vi "HFRR ADV v036 new software.vi"() -> ()   [LabVIEW 2025] (continued)
          tunnel: [T19."Disabled" ("Disabled") T19."Enabled" ("Disabled")] -> w1363
          frame False {
          }
          frame True {
          }
        }
        n1483 = property on="About" class="Bool (strict)"("DisabledEnum"=w1363) -> ()  [unwired: 2 in, 2 out]
      }
      frame "Test Setup" {
        w1369 = T19."Enabled" ("Disabled")
        n1484 = local read "Service Password enable"() -> (w1368:bool)
        n1485 = property on="Dashboard" class="Bool (strict)"("DisabledEnum"=T19."Disabled" ("Disabled")) -> ()  [unwired: 2 in, 2 out]
        n1486 = property on="Imaging" class="Bool (strict)"("DisabledEnum"=w1369) -> ()  [unwired: 2 in, 2 out]
        n1487 = property on="Analysis" class="Bool (strict)"("DisabledEnum"=w1369) -> ()  [unwired: 2 in, 2 out]
        n1488 = property on="Home" class="Bool (strict)"("DisabledEnum"=w1369) -> ()  [unwired: 2 in, 2 out]
        n1489 = property on="Report" class="Bool (strict)"("DisabledEnum"=w1369) -> ()  [unwired: 2 in, 2 out]
        n1490 = property on="Test Setup" class="Bool (strict)"("DisabledEnum"=w1369) -> ()  [unwired: 2 in, 2 out]
        n1491 = case shown="True" w1368 {
          tunnel: [T19."Disabled" ("Disabled") T19."Enabled" ("Disabled")] -> w1367
          frame False {
          }
          frame True {
          }
        }
        n1492 = property on="About" class="Bool (strict)"("DisabledEnum"=w1367) -> ()  [unwired: 2 in, 2 out]
      }
      frame "Adv Scar" {
        w1376 = T19."Enabled" ("Disabled")
        n1493 = property on="Dashboard" class="Bool (strict)"("DisabledEnum"=T19."Disabled" ("Disabled")) -> ()  [unwired: 2 in, 2 out]
        n1494 = property on="Imaging" class="Bool (strict)"("DisabledEnum"=w1376) -> ()  [unwired: 2 in, 2 out]
        n1495 = property on="Analysis" class="Bool (strict)"("DisabledEnum"=w1376) -> ()  [unwired: 2 in, 2 out]
        n1496 = property on="Home" class="Bool (strict)"("DisabledEnum"=w1376) -> ()  [unwired: 2 in, 2 out]
        n1497 = property on="Report" class="Bool (strict)"("DisabledEnum"=w1376) -> ()  [unwired: 2 in, 2 out]
        n1498 = property on="Test Setup" class="Bool (strict)"("DisabledEnum"=w1376) -> ()  [unwired: 2 in, 2 out]
        n1499 = local read "Service Password enable"() -> (w1374:bool)
        n1500 = case shown="True" w1374 {
          tunnel: [T19."Disabled" ("Disabled") T19."Enabled" ("Disabled")] -> w1373
          frame False {
          }
          frame True {
          }
        }
        n1501 = property on="About" class="Bool (strict)"("DisabledEnum"=w1373) -> ()  [unwired: 2 in, 2 out]
      }
      frame "Calibration" {
        w1379 = T19."Enabled" ("Disabled")
        n1502 = property on="Dashboard" class="Bool (strict)"("DisabledEnum"=T19."Disabled" ("Disabled")) -> ()  [unwired: 2 in, 2 out]
        n1503 = property on="Imaging" class="Bool (strict)"("DisabledEnum"=w1379) -> ()  [unwired: 2 in, 2 out]
        n1504 = property on="Analysis" class="Bool (strict)"("DisabledEnum"=w1379) -> ()  [unwired: 2 in, 2 out]
        n1505 = property on="Home" class="Bool (strict)"("DisabledEnum"=w1379) -> ()  [unwired: 2 in, 2 out]
        n1506 = property on="Report" class="Bool (strict)"("DisabledEnum"=w1379) -> ()  [unwired: 2 in, 2 out]
        n1507 = property on="Test Setup" class="Bool (strict)"("DisabledEnum"=w1379) -> ()  [unwired: 2 in, 2 out]
        n1508 = local read "Service Password enable"() -> (w1381:bool)
        n1509 = property on="Calibration" class="Bool (strict)"("DisabledEnum"=w1379) -> ()  [unwired: 2 in, 2 out]
        n1510 = case shown="True" w1381 {
          tunnel: [T19."Disabled" ("Disabled") T19."Enabled" ("Disabled")] -> w1380
          frame False {
          }
          frame True {
          }
        }
        n1511 = property on="About" class="Bool (strict)"("DisabledEnum"=w1380) -> ()  [unwired: 2 in, 2 out]
      }
      frame "Adv Scar Report" {
        w1387 = T19."Enabled" ("Disabled")
        n1512 = property on="Dashboard" class="Bool (strict)"("DisabledEnum"=T19."Disabled" ("Disabled")) -> ()  [unwired: 2 in, 2 out]
        n1513 = property on="Imaging" class="Bool (strict)"("DisabledEnum"=w1387) -> ()  [unwired: 2 in, 2 out]
        n1514 = property on="Analysis" class="Bool (strict)"("DisabledEnum"=w1387) -> ()  [unwired: 2 in, 2 out]
        n1515 = property on="Home" class="Bool (strict)"("DisabledEnum"=w1387) -> ()  [unwired: 2 in, 2 out]
        n1516 = property on="Report" class="Bool (strict)"("DisabledEnum"=w1387) -> ()  [unwired: 2 in, 2 out]
        n1517 = property on="Test Setup" class="Bool (strict)"("DisabledEnum"=w1387) -> ()  [unwired: 2 in, 2 out]
        n1518 = local read "Service Password enable"() -> (w1386:bool)
        n1519 = case shown="True" w1386 {
          tunnel: [T19."Disabled" ("Disabled") T19."Enabled" ("Disabled")] -> w1385
          frame False {
          }
          frame True {
          }
        }
        n1520 = property on="About" class="Bool (strict)"("DisabledEnum"=w1385) -> ()  [unwired: 2 in, 2 out]
      }
      frame "Compare Files" {
        w1393 = T19."Enabled" ("Disabled")
        n1521 = local read "Service Password enable"() -> (w1392:bool)
        n1522 = property on="Dashboard" class="Bool (strict)"("DisabledEnum"=T19."Disabled" ("Disabled")) -> ()  [unwired: 2 in, 2 out]
        n1523 = property on="Imaging" class="Bool (strict)"("DisabledEnum"=w1393) -> ()  [unwired: 2 in, 2 out]
        n1524 = property on="Analysis" class="Bool (strict)"("DisabledEnum"=w1393) -> ()  [unwired: 2 in, 2 out]
        n1525 = property on="Home" class="Bool (strict)"("DisabledEnum"=w1393) -> ()  [unwired: 2 in, 2 out]
        n1526 = property on="Report" class="Bool (strict)"("DisabledEnum"=w1393) -> ()  [unwired: 2 in, 2 out]
        n1527 = property on="Test Setup" class="Bool (strict)"("DisabledEnum"=w1393) -> ()  [unwired: 2 in, 2 out]
        n1528 = case shown="True" w1392 {
          tunnel: [T19."Disabled" ("Disabled") T19."Enabled" ("Disabled")] -> w1391
          frame False {
          }
          frame True {
          }
        }
        n1529 = property on="About" class="Bool (strict)"("DisabledEnum"=w1391) -> ()  [unwired: 2 in, 2 out]
      }
      frame "Acquire" {
        n1530 = local read "Service Password enable"() -> (w1398:bool)
        n1531 = property on="Test Setup" class="Bool (strict)"("DisabledEnum"=T19."Disabled" ("Disabled")) -> ()  [unwired: 2 in, 2 out]
        n1532 = local read "Auto Start Test"() -> (w1400:bool)
        n1533 = local read "RUN"() -> (w1402:bool)
        n1534 = case shown="True" w1398 {
          tunnel: [T19."Disabled" ("Disabled") T19."Enabled" ("Disabled")] -> w1399
          frame False {
          }
          frame True {
          }
        }
        n1535 = Or(x=w1402, y=w1400) -> (x .or. y?=w1401:bool)
        n1536 = case shown="True" w1401 {
          tunnel: [T19."Enabled" ("Disabled") T19."Disabled" ("Disabled")] -> w1397
          frame False {
          }
          frame True {
          }
        }
        n1537 = property on="About" class="Bool (strict)"("DisabledEnum"=w1399) -> ()  [unwired: 2 in, 2 out]
        n1538 = property on="Imaging" class="Bool (strict)"("DisabledEnum"=w1397) -> ()  [unwired: 2 in, 2 out]
        n1539 = property on="Dashboard" class="Bool (strict)"("DisabledEnum"=w1397) -> ()  [unwired: 2 in, 2 out]
        n1540 = property on="Analysis" class="Bool (strict)"("DisabledEnum"=w1397) -> ()  [unwired: 2 in, 2 out]
        n1541 = property on="Home" class="Bool (strict)"("DisabledEnum"=w1397) -> ()  [unwired: 2 in, 2 out]
        n1542 = property on="Report" class="Bool (strict)"("DisabledEnum"=w1397) -> ()  [unwired: 2 in, 2 out]
        n1543 = property on="Calibration" class="Bool (strict)"("DisabledEnum"=w1397) -> ()  [unwired: 2 in, 2 out]
      }
      frame "About" {
        n1544 = local read "FILE"() -> (w1416:string)
        n1545 = local read "TEST FILE NAM,E SAVED"() -> (w1409:bool)
        n1546 = call <vilib>:"Trim Whitespace.vi"("string"=w1416) -> ("trimmed string"=w1415:string)  [unwired: 1 in]
        n1547 = local read "Auto Start Test"() -> (w1419:bool)
        n1548 = String Length(string=w1415) -> (length=w1414:i32)
        n1549 = Greater?(x=w1414, y=1) -> (0:w1411:bool)
        n1550 = And(x=w1411, y=w1409) -> (x .and. y?=w1410:bool)
        n1551 = local read "RUN"() -> (w1421:bool)
        n1552 = case shown="True" w1410 {
          tunnel: [T19."Disabled" ("Disabled") T19."Enabled" ("Disabled")] -> w1412
          frame False {
          }
          frame True {
          }
        }
        n1553 = Or(x=w1421, y=w1419) -> (x .or. y?=w1420:bool)
        n1554 = property on="About" class="Bool (strict)"("DisabledEnum"=T19."Enabled" ("Disabled")) -> ()  [unwired: 2 in, 2 out]
        n1555 = case shown="False" w1420 {
          tunnel: [T19."Enabled" ("Disabled") T19."Disabled" ("Disabled")] -> w1418
          frame False {
          }
          frame True {
          }
        }
        n1556 = property on="Dashboard" class="Bool (strict)"("DisabledEnum"=w1412) -> ()  [unwired: 2 in, 2 out]
        n1557 = property on="Test Setup" class="Bool (strict)"("DisabledEnum"=T19."Disabled" ("Disabled")) -> ()  [unwired: 2 in, 2 out]
        n1558 = property on="Imaging" class="Bool (strict)"("DisabledEnum"=w1418) -> ()  [unwired: 2 in, 2 out]
        n1559 = property on="Analysis" class="Bool (strict)"("DisabledEnum"=w1418) -> ()  [unwired: 2 in, 2 out]
        n1560 = property on="Home" class="Bool (strict)"("DisabledEnum"=w1418) -> ()  [unwired: 2 in, 2 out]
        n1561 = property on="Report" class="Bool (strict)"("DisabledEnum"=w1418) -> ()  [unwired: 2 in, 2 out]
      }
    }
    n1562 = local read "Quit"() -> (w1346:bool)
    "Single" <- "Single - Graph"
  }
  n1563 = disable-structure shown="Disabled" {
    disable-tunnel: [w1699 _] -> w42
    disable-tunnel: _ -> [w1698 _]
    frame Disabled {
      n1564 = while {
        tunnel: w1698 -> [_]
        tunnel: [w1700] -> w1699
        tunnel: [w1701] -> _
        i -> [w1701]
        stop <- w1700 stop-if-true
        w1717 = u16 10 items=["1.0"=10, "1.5"=15, "2.0"=20] ("stop bits (10: 1 bit)")
        n1565 = Wait (ms)(milliseconds to wait=u32 10) -> ()  [unwired: 1 out]
        n1566 = call-poly "VISA Configure Serial Port"("VISA resource name"=refnum<visa-resource-name> "ASRL1::INSTR" ("COM PORT"), "timeout (10sec)"=u32 10, "baud rate (9600)"=u32 57600, "data bits (8)"=u16 8, "stop bits (10: 1 bit)"=w1717) -> ("VISA resource name out"=w1703:refnum<visa-resource-name>, "error out"=w1712:errorcluster)  [unwired: 9 in]
        n1567 = VISA Read(VISA resource name=w1703, byte count=u32 2 ("byte count (0)")) -> (read buffer=w1711:string)  [unwired: 1 in, 3 out]
        n1568 = String Subset(string=w1711, offset (0)=0, length (rest)=2 ("length (rest)")) -> (substring=w1710:string)
        n1569 = Match Pattern(string=w1710, regular expression="<>") -> (offset past match=w1707:i32)  [unwired: 1 in, 3 out]
        n1570 = Greater Or Equal?(x=w1707, y=0) -> (x >= y?=w1702:bool)
        n1571 = case shown="True" w1702 {
          tunnel: w1703 -> [_ w1721]
          tunnel: w1712 -> [_ w1720]
          frame False {
          }
          frame True {
            n1572 = VISA Read(VISA resource name=w1721, byte count=u32 32 ("byte count (0)"), error in (no error)=w1720) -> (read buffer=w1719:string)  [unwired: 3 out]
            n1573 = String Subset(string=w1719, offset (0)=0, length (rest)=8 ("length (rest)")) -> (substring=w1723:string)
            n1574 = String Subset(string=w1719, offset (0)=8, length (rest)=8 ("length (rest)")) -> (substring=w1724:string)
            n1575 = Decimal String To Number(string=w1724) -> (number=w1731:i32)  [unwired: 2 in, 1 out]
            n1576 = Decimal String To Number(string=w1723) -> (number=w1727:i32)  [unwired: 2 in, 1 out]
            n1577 = Divide(x=w1731, y=10000) -> ()  [unwired: 1 out]
            n1578 = Divide(x=w1727, y=1000000) -> ()  [unwired: 1 out]
          }
        }
        n1579 = local read "Quit"() -> (w1700:bool)
      }
    }
    frame Enabled {
    }
  }
  n1580 = Tick Count (ms)() -> (millisecond timer value=w4:u32)
  n1581 = while {
    shift-right: [w1777] -> _
    shift-left: w6 -> [w1781]
    shift-right: [w1776] -> _
    shift-left: w5 -> [w1780]
    shift-right: [w1775] -> _
    shift-left: w6 -> [w1779]
    shift-right: [w1774] -> _
    shift-left: w5 -> [w1778]
    shift-right: [w1772] -> _
    shift-left: w4 -> [w1773]
    shift-right: [w1769] -> _
    shift-left: w3 -> [w1770]
    shift-right: [w1768] -> _
    shift-left: w3 -> [w1771]
    shift-right: [w1761] -> _
    shift-left: w3 -> [w1767]
    shift-right: [w1760] -> _
    shift-left: w3 -> [w1766]
    shift-right: [w1759] -> _
    shift-left: w3 -> [w1765]
    shift-right: [w1758] -> _
    shift-left: w3 -> [w1764]
    shift-right: [w1757] -> _
    shift-left: w3 -> [w1763]
    shift-right: [w1756] -> _
    shift-left: w3 -> [w1762]
    shift-right: [w1755] -> _
    shift-left: w3 -> [w1749]
    shift-right: [w1754] -> _
    shift-left: w3 -> [w1748]
    shift-right: [w1753] -> _
    shift-left: w3 -> [w1747]
    shift-right: [w1752] -> _
    shift-left: w3 -> [w1746]
    shift-right: [w1751] -> _
    shift-left: w3 -> [w1745]
    shift-right: [w1750] -> _
    shift-left: w3 -> [w1744]
    shift-right: [w1735] -> _
    shift-left: w3 -> [w1738]
    shift-right: [w1734] -> _
    shift-left: w3 -> [w1737]
    shift-right: [w1733] -> _
    shift-left: w3 -> [w1736]
    stop <- w1783 stop-if-true
    n1582 = local read "Read UNO"() -> (w1742:string)
    n1583 = local read "Error  2"() -> (w1782:errorcluster)
    n1584 = String Length(string=w1742) -> (length=w1741:i32)
    n1585 = call <vilib>:"Trim Whitespace.vi"("string"=w1742) -> ("trimmed string"=w1743:string)  [unwired: 1 in]
    n1586 = Greater Or Equal?(x=w1741, y=23) -> (x >= y?=w1739:bool)
    n1587 = case shown="No Error" w1782 {
      tunnel: w1781 -> [w1829 w1925]
      tunnel: w1780 -> [w1828 w1924]
      tunnel: w1779 -> [w1827 w1923]
      tunnel: w1778 -> [w1826 w1922]
      tunnel: [w1825 w1925] -> w1777
      tunnel: [w1824 w1924] -> w1776
      tunnel: [w1823 w1923] -> w1775
      tunnel: [w1822 w1922] -> w1774
      tunnel: w1773 -> [w1821 w1921]
      tunnel: [w1820 w1921] -> w1772
      tunnel: w1770 -> [w1819 w1920]
      tunnel: w1771 -> [w1818 w1919]
      tunnel: [w1817 w1920] -> w1769
      tunnel: [w1816 w1919] -> w1768
      tunnel: w1767 -> [w1815 w1918]
      tunnel: w1766 -> [w1814 w1917]
      tunnel: w1765 -> [w1813 w1916]
      tunnel: w1764 -> [w1812 w1915]
      tunnel: w1763 -> [w1811 w1914]
      tunnel: w1762 -> [w1810 w1913]
      tunnel: [w1809 w1918] -> w1761
      tunnel: [w1808 w1917] -> w1760
      tunnel: [w1807 w1916] -> w1759
      tunnel: [w1806 w1915] -> w1758
      tunnel: [w1805 w1914] -> w1757
      tunnel: [w1804 w1913] -> w1756
      tunnel: w1749 -> [w1803 w1912]
      tunnel: [w1802 w1912] -> w1755
      tunnel: [w1801 w1908] -> w1754
      tunnel: [w1800 w1907] -> w1753
      tunnel: [w1799 w1911] -> w1752
      tunnel: [w1798 w1910] -> w1751
      tunnel: [w1797 w1909] -> w1750
      tunnel: w1748 -> [w1796 w1911]
      tunnel: w1747 -> [w1795 w1910]
      tunnel: w1746 -> [w1794 w1909]
      tunnel: w1745 -> [w1793 w1908]
      tunnel: w1744 -> [w1792 w1907]
      tunnel: w1743 -> [w1791 _]
      tunnel: w1739 -> [w1790 _]
      tunnel: w1738 -> [w1789 w1906]
      tunnel: w1737 -> [w1788 w1905]
      tunnel: w1736 -> [w1787 w1904]
      tunnel: [w1786 w1906] -> w1735
      tunnel: [w1785 w1905] -> w1734
      tunnel: [w1784 w1904] -> w1733
      frame No Error {
        n1588 = case shown="True" w1790 {
          tunnel: w1829 -> [w1845 w1897]
          tunnel: w1828 -> [w1844 w1896]
          tunnel: w1827 -> [w1843 w1895]
          tunnel: w1826 -> [w1842 w1894]
          tunnel: [w1845 w1893] -> w1825
          tunnel: [w1844 w1892] -> w1824
          tunnel: [w1843 w1891] -> w1823
          tunnel: [w1842 w1890] -> w1822
          tunnel: w1821 -> [w1841 w1888]
          tunnel: [w1841 w1887] -> w1820
          tunnel: w1819 -> [w1840 w1886]
          tunnel: w1818 -> [w1839 w1885]
          tunnel: [w1840 w1884] -> w1817
          tunnel: [w1839 w1883] -> w1816
          tunnel: w1815 -> [w1838 w1882]
          tunnel: w1814 -> [w1837 w1881]
          tunnel: w1813 -> [w1836 w1880]
          tunnel: w1812 -> [w1835 w1879]
          tunnel: w1811 -> [w1834 w1878]
          tunnel: w1810 -> [w1833 w1877]
          tunnel: [w1838 w1876] -> w1809
          tunnel: [w1837 w1875] -> w1808
          tunnel: [w1836 w1874] -> w1807
          tunnel: [w1835 w1873] -> w1806
          tunnel: [w1834 w1872] -> w1805
          tunnel: [w1833 w1871] -> w1804
          tunnel: w1803 -> [w1851 w1870]
          tunnel: [w1851 w1869] -> w1802
          tunnel: [w1848 w1868] -> w1801
          tunnel: [w1847 w1867] -> w1800
          tunnel: [w1850 w1866] -> w1799
          tunnel: [w1846 w1865] -> w1798
          tunnel: [w1849 w1864] -> w1797
          tunnel: w1796 -> [w1850 w1863]
          tunnel: w1795 -> [w1849 w1862]
          tunnel: w1794 -> [w1848 w1861]
          tunnel: w1793 -> [w1847 w1860]
          tunnel: w1792 -> [w1846 w1859]
          tunnel: w1791 -> [_ w1858]
          tunnel: w1789 -> [w1832 w1857]
          tunnel: w1788 -> [w1831 w1856]
          tunnel: w1787 -> [w1830 w1855]
          tunnel: [w1832 w1854] -> w1786
          tunnel: [w1831 w1853] -> w1785
          tunnel: [w1830 w1852] -> w1784
          frame False {
          }
          frame True {
            n1589 = Tick Count (ms)() -> (millisecond timer value=w1889:u32)
            n1590 = String To Byte Array(string=w1858) -> (unsigned byte array=w1902:u8[])
            n1591 = Array Size(array=w1902) -> (size(s)=w1901:i32)
            n1592 = formula code="// --- INTERNAL VARIABLE DECLARATIONS ---\nint i = 0;\nint k = 0;\nint start_idx = -1;\nint end_idx = -1;\nint phase = 0;\nint sign0 = 1;\nint sign1 = 1;\nint ch0_val = 0;   \nint ch1_val = 0;   \nfloat ch0_raw = 0.0;\nfloat ch1_raw = 0.0;\nfloat temp0 = 0.0;\nfloat temp1 = 0.0;\nfloat ch0_clean = 0.0;\nfloat ch1_clean = 0.0;\n\nint valid_samples = 0; // FIX: Track if we actually parsed new data this window\nfloat max_allowed_bits = 8388607.0; // FIX: Change this to match your ADC max value\n\n// Temporal intermediate variables for calculation smoothing\nfloat raw_p2p_v = 0.0;\nfloat raw_friction = 0.0;\nfloat raw_cof = 0.0;\n\n// Temporal intermediate variables for Piezo voltage translations\nfloat piezo_min_v = 0.0;\nfloat piezo_max_v = 0.0;\n\n// Initialize output variables to current shift register states right away\nout_LVDT_Min_V = in_LVDT_Min_V;\nout_LVDT_Max_V = in_LVDT_Max_V;\nout_LVDT_P2P_V = in_LVDT_P2P_V;\nout_Piezo_P2P = in_Piezo_P2P;\nout_Friction_N = in_Friction_N;\nout_COF = in_COF;\nwindow_ready = 0;\n\n// --- STEP 1: PARSE EVERY STRING IN THE BYTE ARRAY ---\nif (array_size > 2) {\n    for (i = 0; i < array_size - 1; i++) {\n        if (raw_bytes[i] == 42) { // '*' character detected\n            start_idx = i;\n        }\n        \n        // Match standard delimiter sequence \";&\" or end window character\n        if (raw_bytes[i] == 59 && raw_bytes[i+1] == 38 && start_idx != -1) { \n            end_idx = i;\n            ch0_val = 0;\n            ch1_val = 0;\n            sign0 = 1;\n            sign1 = 1;\n            phase = 0; \n\n            for (k = start_idx + 1; k < end_idx; k++) {\n                if (raw_bytes[k] == 45) { // '-' sign\n                    if (phase == 0) sign0 = -1;\n                    else sign1 = -1;\n                }\n                else if (raw_bytes[k] == 43) { // '+' sign\n                    if (phase == 0) sign0 = 1;\n                    else sign1 = 1;\n                }\n                else if (raw_bytes[k] == 59) { // ';' delimiter\n                    phase = 1; \n                }\n                else if (raw_bytes[k] >= 48 && raw_bytes[k] <= 57) { // Numeric ASCII digits\n                    if (phase == 0) {\n                        ch0_val = (ch0_val * 10) + (raw_bytes[k] - 48);\n                    } else {\n                        ch1_val = (ch1_val * 10) + (raw_bytes[k] - 48);\n                    }\n                }\n            }\n\n            // Implicit type conversion\n            ch0_raw = ch0_val * sign0 * 1.0;\n            ch1_raw = ch1_val * sign1 * 1.0;\n\n            // FIX: Sanity check / Hard-clamping to catch sudden massive ASCII noise spikes\n            if (ch0_raw > max_allowed_bits)  ch0_raw = max_allowed_bits;\n            if (ch0_raw < -max_allowed_bits) ch0_raw = -max_allowed_bits;\n            if (ch1_raw > max_allowed_bits)  ch1_raw = max_allowed_bits;\n            if (ch1_raw < -max_allowed_bits) ch1_raw = -max_allowed_bits;\n\n            // --- STEP 2: 3-SAMPLE MEDIAN FILTER ---\n            m0_2 = m0_1; m0_1 = m0_0; m0_0 = ch0_raw;\n            float s0_0 = m0_0; float s0_1 = m0_1; float s0_2 = m0_2;\n            if (s0_0 > s0_1) { temp0 = s0_0; s0_0 = s0_1; s0_1 = temp0; }\n            if (s0_1 > s0_2) { temp0 = s0_1; s0_1 = s0_2; s0_2 = temp0; }\n            if (s0_0 > s0_1) { temp0 = s0_0; s0_0 = s0_1; s0_1 = temp0; }\n            ch0_clean = s0_1;\n\n            m1_2 = m1_1; m1_1 = m1_0; m1_0 = ch1_raw;\n            float s1_0 = m1_0; float s1_1 = m1_1; float s1_2 = m1_2;\n            if (s1_0 > s1_1) { temp1 = s1_0; s1_0 = s1_1; s1_1 = temp1; }\n            if (s1_1 > s1_2) { temp1 = s1_1; s1_1 = s1_2; s1_2 = temp1; }\n            if (s1_0 > s1_1) { temp1 = s1_0; s1_0 = s1_1; s1_1 = temp1; }\n            ch1_clean = s1_1;\n\n            // --- STEP 3: EXPONENTIAL FILTER (STREAM LEVEL) ---\n            if (ch0_filt == 0.0) ch0_filt = ch0_clean;\n            if (ch1_filt == 0.0) ch1_filt = ch1_clean;\n\n            ch0_filt = ch0_filt + (ch0_clean - ch0_filt) * 0.125;\n            ch1_filt = ch1_filt + (ch1_clean - ch1_filt) * 0.125;\n\n            // --- STEP 4: MIN/MAX WINDOW CONTINUOUS ACCUMULATION ---\n            if (ch0_filt > max_ch0) max_ch0 = ch0_filt;\n            if (ch0_filt < min_ch0) min_ch0 = ch0_filt;\n            if (ch1_filt > max_ch1) max_ch1 = ch1_filt;\n            if (ch1_filt < min_ch1) min_ch1 = ch1_filt;\n\n            valid_samples++; // FIX: Successfully parsed and accumulated a clean point\n            start_idx = -1; \n        }\n    }\n}\n\n// --- STEP 5: WINDOW EVALUATION ENGINE ---\n// FIX: Condition updated to verify that valid samples exist for both channels\nif (((current_time_ms - start_time_ms) >= 50) && (valid_samples > 0) && (min_ch0 < 9000000.0) && (min_ch1 < 9000000.0)) {\n    window_ready = 1;\n\n    // Linear Bit-to-Voltage Transformations (LVDT - Channel 0)\n    out_LVDT_Min_V = (min_ch0 * VREF) / 8388607.0;\n    out_LVDT_Max_V = (max_ch0 * VREF) / 8388607.0;\n    raw_p2p_v = out_LVDT_Max_V - out_LVDT_Min_V;\n\n    // Linear Bit-to-Voltage Transformations (Piezo - Channel 1)\n    piezo_min_v = (min_ch1 * VREF) / 8388607.0;\n    piezo_max_v = (max_ch1 * VREF) / 8388607.0;\n    \n    // Assign Peak-to-Peak Voltage directly to output indicator (Matches Python logic)\n    out_Piezo_P2P = piezo_max_v - piezo_min_v;\n    \n    // Force scaling calculations using Voltage delta * Newtons/Volt Factor\n    raw_friction = out_Piezo_P2P * PIEZO_CAL_FACTOR + 0.44528;\n    raw_cof = raw_friction / NORMAL_FORCE;\n\n    // --- STEP 6: OUTPUT METRIC SMOOTHING (Low-Pass Filter Alpha = 0.05) ---\n    // Seed initial historical metrics if first loop iteration\n    if (hist_LVDT_P2P == 0.0) hist_LVDT_P2P = raw_p2p_v;\n    if (hist_Friction == 0.0) hist_Friction = raw_friction;\n    if (hist_COF == 0.0)      hist_COF = raw_cof;\n\n    // Apply exponential output dampening\n    hist_LVDT_P2P = hist_LVDT_P2P + (raw_p2p_v - hist_LVDT_P2P) * 0.05;\n    hist_Friction = hist_Friction + (raw_friction - hist_Friction) * 0.05; // Note: Can drop to 0.02 for more aggressive damping\n    hist_COF      = hist_COF + (raw_cof - hist_COF) * 0.05;\n\n    // Direct smoothed parameters out to UI Indicators\n    out_LVDT_P2P_V = hist_LVDT_P2P;\n    out_Friction_N = hist_Friction;\n    out_COF        = hist_COF;\n\n    // Reset tracking targets to extreme boundaries safely\n    min_ch0 = 9999999.0;\n    max_ch0 = -9999999.0;\n    min_ch1 = 9999999.0;\n    max_ch1 = -9999999.0;\n\n    valid_samples = 0; // FIX: Reset counter for next time frame\n    start_time_ms = current_time_ms;\n}"("raw_bytes"=w1902, "array_size"=w1901, "VREF"="VREF", "PIEZO_CAL_FACTOR"="PIEZO_CAL_FACTOR", "NORMAL_FORCE"="NORMAL_FORCE", "min_ch0"=w1897, "max_ch0"=w1896, "min_ch1"=w1895, "max_ch1"=w1894, "current_time_ms"=w1889, "start_time_ms"=w1888, "ch0_filt"=w1886, "ch1_filt"=w1885, "m0_0"=w1882, "m0_1"=w1881, "m0_2"=w1880, "m1_0"=w1879, "m1_1"=w1878, "m1_2"=w1877, "in_LVDT_Min_V"=w1870, "in_LVDT_Max_V"=w1863, "in_LVDT_P2P_V"=w1862, "in_Piezo_P2P"=w1861, "in_Friction_N"=w1860, "in_COF"=w1859, "hist_LVDT_P2P"=w1857, "hist_Friction"=w1856, "hist_COF"=w1855) -> ("window_ready"=→"Valid_data":dbl, "out_LVDT_Min_V"=w1869:dbl, "out_LVDT_Max_V"=w1868:dbl, "out_LVDT_P2P_V"=w1867:dbl, "out_Piezo_P2P"=w1866:dbl, "out_Friction_N"=w1865:dbl, "out_COF"=w1864:dbl, "min_ch0"=w1893:dbl, "max_ch0"=w1892:dbl, "min_ch1"=w1891:dbl, "max_ch1"=w1890:dbl, "start_time_ms"=w1887:u32, "ch0_filt"=w1884:dbl, "ch1_filt"=w1883:dbl, "m0_0"=w1876:dbl, "m0_1"=w1875:dbl, "m0_2"=w1874:dbl, "m1_0"=w1873:dbl, "m1_1"=w1872:dbl, "m1_2"=w1871:dbl, "hist_LVDT_P2P"=w1854:dbl, "hist_Friction"=w1853:dbl, "hist_COF"=w1852:dbl)
            "LVDT MIN" <- w1869
            "LVDT MAX" <- w1868
            "LVDT Peak" <- w1867
            "pizo raw" <- w1866
            "cof" <- w1864
            "Frictioin Force Raw" <- w1865
          }
        }
      }
      frame Error {
      }
    }
    n1593 = local read "Quit"() -> (w1783:bool)
  }
  n1594 = disable-structure shown="Disabled" {
    disable-tunnel: errorcluster {"status"=TRUE, "code"=0, "source"="Init"} ("error IO") -> [w1928 _]
    disable-tunnel: [w1926 _] -> w45
    frame Disabled {
      n1595 = while {
        shift-right: [w1944] -> w1930
        shift-left: _ -> [w1935]
        shift-right: [w1943] -> w1929
        shift-left: w1928 -> [w1937]
        tunnel: [w1932] -> w1926
        tunnel: [w1942] -> _
        i -> [w1942]
        stop <- w1932 stop-if-true
        n1596 = local read "Port 1a"() -> (w1938:bool)
        n1597 = local read "Port 3"() -> (w1939:bool)
        n1598 = local read "Com Port 1"() -> (w1936:refnum<visa-resource-name>)
        n1599 = Or(x=w1939, y=w1938) -> (x .or. y?=w1941:bool)
        n1600 = Unbundle(w1937) -> ("status"=→"Port 3":bool)  [unwired: 2 out]
        n1601 = Not Equal?(x=w1936, y=w1935) -> (x != y?=w1933:bool)
        n1602 = case shown="True" w1941 {
          frame False {
            w1947 = TRUE ("Visible")
            n1603 = property on="Port 1a" class="Bool (strict)"("Visible"=w1947) -> ()  [unwired: 2 in, 2 out]
            n1604 = property on="Port 3" class="Bool (strict)"("Visible"=w1947) -> ()  [unwired: 2 in, 2 out]
          }
          frame True {
            w1948 = TRUE ("Visible")
            n1605 = property on="Port 1a" class="Bool (strict)"("Visible"=w1948) -> ()  [unwired: 2 in, 2 out]
            n1606 = property on="Port 3" class="Bool (strict)"("Visible"=w1948) -> ()  [unwired: 2 in, 2 out]
          }
        }
        n1607 = Wait (ms)(milliseconds to wait=u32 40) -> ()  [unwired: 1 out]
        n1608 = case shown="True" w1933 {
          tunnel: [w1945 errorcluster {"status"=TRUE, "code"=0, "source"="Init"} ("error out")] -> w1934
          tunnel: w1937 -> [w1945 _]
          frame False {
          }
          frame True {
          }
        }
        n1609 = case shown="Error" w1934 {
          selector: w1934 -> [w1955 w1973]
          tunnel: [w1958 w1977] -> w1944
          tunnel: [w1957 w1971] -> w1943
          tunnel: w1935 -> [w1956 w1975]
          frame No Error {
            n1610 = property class="Instr"(reference=w1956, error in=w1955) -> (reference out=w1953:refnum<visa-resource-name>, error out=w1954:errorcluster, "Serial Settings:Number of Bytes at Serial Port"=w1950:u32)
            n1611 = Greater?(x=w1950, y=u32 5) -> (0:w1949:bool)
            n1612 = Not(x=w1949) -> (.not. x?=→"Port 1a":bool)
            n1613 = while {
              tunnel: [w1966] -> w1957
              tunnel: [w1965] -> w1958
              tunnel: w1954 -> [w1964]
              tunnel: w1953 -> [w1963]
              stop <- TRUE stop-if-true
              n1614 = property class="Instr" props=["Serial Settings:Number of Bytes at Serial Port"](reference=w1963, error in=w1964) -> (reference out=w1968:refnum<visa-resource-name>, error out=w1967:errorcluster)  [unwired: 1 out]
              n1615 = VISA Read(VISA resource name=w1968, byte count=u32 50, error in (no error)=w1967) -> (VISA resource name out=w1965:refnum<visa-resource-name>, read buffer=w1960:string, error out=w1966:errorcluster)  [unwired: 1 out]
              n1616 = Wait (ms)(milliseconds to wait=u32 5) -> ()  [unwired: 1 out]
            }
          }
          frame Error {
            w1983 = u16 0 items=["None", "XON/XOFF", "RTS/CTS", "XON/XOFF & RTS/CTS", "DTR/DSR", "XON/XOFF & DTR/DSR"] ("flow control (0:none)  2")
            w1981 = u16 10 items=["1.0"=10, "1.5"=15, "2.0"=20] ("stop bits 2")
            w1979 = u16 0 items=["None", "Odd", "Even", "Mark", "Space"] ("parity 2")
            w1980 = u32 10000  # timeout (10sec)
            n1617 = VISA Close(VISA resource name=w1975, error in (no error)=w1973) -> (error out=w1976:errorcluster)
            n1618 = local write "Port 1a"(FALSE ("Port 1a")) -> ()
            n1619 = local read "Com Port 1"() -> (w1970:refnum<visa-resource-name>)
            n1620 = call <vilib>:"Clear Errors.vi"("error in (no error)"=w1976) -> ("error out"=w1974:errorcluster)  [unwired: 5 in, 1 out]
            n1621 = call-poly "VISA Configure Serial Port"("VISA resource name"=w1970, "timeout (10sec)"=w1980, "baud rate (9600)"=u32 250000 ("baud rate  2"), "data bits (8)"=u16 8 ("data bits  2"), "parity (0:none)"=w1979, "error in (no error)"=w1974, "stop bits (10: 1 bit)"=w1981, "flow control (0:none)"=w1983) -> ("VISA resource name out"=w1984:refnum<visa-resource-name>, "error out"=w1985:errorcluster)  [unwired: 6 in]
            n1622 = flat-sequence {
              tunnel: w1984 -> [w1987]
              tunnel: w1985 -> [w1986]
              tunnel: [w1987] -> w1977
              tunnel: [w1986] -> w1971
              frame #0 {
                n1623 = Wait (ms)(milliseconds to wait=u32 50) -> ()  [unwired: 1 out]
              }
            }
            "Residual Uno" <- ""
          }
        }
        n1624 = local read "Quit"() -> (w1932:bool)
        "Error Uno" <- w1937
      }
      n1625 = VISA Close(VISA resource name=w1930, error in (no error)=w1929) -> (error out=w1927:errorcluster)
      n1626 = call <vilib>:"Clear Errors.vi"("error in (no error)"=w1927) -> ()  [unwired: 5 in, 2 out]
    }
    frame Enabled {
    }
  }
  n1627 = while {
    stop <- w1998 stop-if-true
    # "V0OLTAGE TO STROKE (peice vise calibration)"
    n1628 = local read "LVDT MIN"() -> (w1990:dbl)
    n1629 = local read "LVDT Peak"() -> (w1989:dbl)
    n1630 = Wait (ms)(milliseconds to wait=u32 10) -> ()  [unwired: 1 out]
    n1631 = formula code="// Dynamic Parameterized Linear Interpolation Node\n// Inputs: vpp_val, voltages (Array), distances (Array)\n// Outputs: stroke\n\nint i = 0;\nint segments = 11; // 12 points make 11 interpolation segments\n\n// 1. Lower Boundary Clamp\nif (vpp_val <= voltages[0]) {\n    stroke = distances[0];\n}\n// 2. Upper Boundary Clamp\nelse if (vpp_val >= voltages[segments]) {\n    stroke = distances[segments];\n}\n// 3. Dynamic Segment Search Loop\nelse {\n    stroke = distances[0]; // Fallback baseline\n    for (i = 0; i < segments; i++) {\n        if (vpp_val >= voltages[i] && vpp_val <= voltages[i+1]) {\n            // Standard linear interpolation formula using array lookups\n            stroke = distances[i] + (vpp_val - voltages[i]) * (distances[i+1] - distances[i]) / (voltages[i+1] - voltages[i]);\n            break; // Segment found, safely exit the loop\n        }\n    }\n}"("vpp_val"=w1989, "voltages"="calibration values", "distances"="STROKE") -> ("stroke"=→"LVDT STROKE":dbl)
    n1632 = local read "Calibration Tare Value"() -> (w1994:dbl)
    n1633 = local read "Calibration Tare"() -> (w1992:bool)
    n1634 = Subtract(x=w1990, y=w1994) -> (x-y=→"LVDT STROKE  Calibration":dbl)
    n1635 = case shown="True" w1992 {
      selector: w1992 -> [_ w2000]
      tunnel: w1990 -> [_ w2001]
      frame False {
      }
      frame True {
        n1636 = Not(x=w2000) -> (.not. x?=w1999:bool)
        n1637 = local write "Calibration Tare"(w1999) -> ()
        "Calibration Tare Value" <- w2001
      }
    }
    n1638 = local read "Quit"() -> (w1998:bool)
  }
  n1639 = while {
    stop <- w2024 stop-if-true
    n1640 = local read "Due read"() -> (w2022:string)
    n1641 = call <vilib>:"High Resolution Polling Wait.vi"("seconds to wait"=0.02) -> ()  [unwired: 10 in, 1 out]
    n1642 = local read "Frictioin Force Raw"() -> (w2004:dbl)
    n1643 = Spreadsheet String To Array(delimiter (Tab)=";", format string="", spreadsheet string=w2022, array type (2D Dbl)=string[] []) -> (array=w2019:string[])
    n1644 = Fract/Exp String To Number(string=w2019) -> (number=w2018:dbl[])  [unwired: 3 in, 1 out]
    n1645 = call <vilib>:"Median Filter PtByPt.vi"("rank"=2, "x"=w2004) -> ("Filtered x"=→"Friction":dbl)  [unwired: 2 in, 1 out]
    n1646 = Index Array(array=w2018) -> (element #1=→"Sample Temperature":dbl, element #2=→"Target Sample Temperature":dbl, element #3=→"Current Duty Cycle":dbl, element #4=→"Ambient Temperature":dbl, element #5=→"Dac Status":dbl, element #6=→"Vpp":dbl, element #7=→"Active Error Code":dbl, element #8=→"Kp":dbl, element #9=→"Ki":dbl, element #10=→"Kd":dbl, element #11=→"SampleRaw":dbl, element #12=→"AmbRaw":dbl)  [unwired: 12 in]
    n1647 = local read "Quit"() -> (w2024:bool)
  }
  n1648 = while {
    shift-right: [w2038] -> w41
    shift-left: _ -> [w2030]
    shift-right: [w2025] -> w40
    shift-left: errorcluster {"status"=FALSE, "code"=0, "source"="Init"} ("error out") -> [w2032]
    tunnel: [w2027] -> w44
    tunnel: [w2037] -> _
    i -> [w2037]
    stop <- w2027 stop-if-true
    n1649 = local read "Com Port 2"() -> (w2031:refnum<visa-resource-name>)
    n1650 = local read "Port 2a"() -> (w2033:bool)
    n1651 = Unbundle(w2032) -> ("status"=→"Port 4":bool)  [unwired: 2 out]
    n1652 = call <vilib>:"High Resolution Polling Wait.vi"("seconds to wait"=0.02) -> ()  [unwired: 10 in, 1 out]
    n1653 = local read "Port 4"() -> (w2034:bool)
    n1654 = Not Equal?(x=w2031, y=w2030) -> (x != y?=w2029:bool)
    n1655 = Or(x=w2034, y=w2033) -> (x .or. y?=w2036:bool)
    n1656 = case shown="False" w2036 {
      frame False {
        w2041 = TRUE ("Visible")
        n1657 = property on="Port 2a" class="Bool (strict)"("Visible"=w2041) -> ()  [unwired: 2 in, 2 out]
        n1658 = property on="Port 4" class="Bool (strict)"("Visible"=w2041) -> ()  [unwired: 2 in, 2 out]
      }
      frame True {
        w2042 = TRUE ("Visible")
        n1659 = property on="Port 2a" class="Bool (strict)"("Visible"=w2042) -> ()  [unwired: 2 in, 2 out]
        n1660 = property on="Port 4" class="Bool (strict)"("Visible"=w2042) -> ()  [unwired: 2 in, 2 out]
      }
    }
    n1661 = case shown="True" w2029 {
      tunnel: [w2039 errorcluster {"status"=TRUE, "code"=0, "source"="Init"} ("error out")] -> w2028
      tunnel: w2032 -> [w2039 _]
      frame False {
      }
      frame True {
      }
    }
    n1662 = case shown="No Error" w2028 {
      selector: w2028 -> [w2055 w2086]
      tunnel: [w2048 w2091] -> w2038
      tunnel: [w2056 w2084] -> w2025
      tunnel: w2030 -> [w2057 w2089]
      frame No Error {
        n1663 = property class="Instr" props=["Serial Settings:Number of Bytes at Serial Port"](reference=w2057, error in=w2055) -> (reference out=w2049:refnum<visa-resource-name>, error out=w2054:errorcluster)  [unwired: 1 out]
        n1664 = while {
          tunnel: [w2065] -> w2050
          tunnel: [w2064] -> w2051
          tunnel: w2054 -> [w2063]
          tunnel: w2049 -> [w2062]
          tunnel: [w2061] -> _
          i -> [w2061]
          stop <- TRUE stop-if-true
          n1665 = property class="Instr" props=["Serial Settings:Number of Bytes at Serial Port"](reference=w2062, error in=w2063) -> (reference out=w2067:refnum<visa-resource-name>, error out=w2066:errorcluster)  [unwired: 1 out]
          n1666 = VISA Read(VISA resource name=w2067, byte count=u32 1000, error in (no error)=w2066) -> (VISA resource name out=w2064:refnum<visa-resource-name>, read buffer=→"Due read":string, error out=w2065:errorcluster)  [unwired: 1 out]
        }
        n1667 = local read "Due Write"() -> (w2047:string)
        n1668 = call <vilib>:"Trim Whitespace.vi"("string"=w2047) -> ("trimmed string"=w2046:string)  [unwired: 1 in]
        n1669 = Not Equal?(x=w2046, y="") -> (x != y?=w2052:bool)
        n1670 = VISA Flush I/O Buffer(VISA resource name=w2051) -> (VISA resource name out=w2044:refnum<visa-resource-name>, error out=→"error out 10":errorcluster)  [unwired: 2 in]
        n1671 = case shown="True" w2052 {
          tunnel: w2044 -> [w2069 w2074]
          tunnel: [w2069 w2078] -> w2048
          tunnel: w2050 -> [w2068 w2073]
          tunnel: [w2068 w2076] -> w2056
          tunnel: w2046 -> [_ w2072]
          tunnel: [_ w2075] -> _
          frame False {
            # "DATA  WRITE LOOP"
          }
          frame True {
            n1672 = Concatenate Strings(w2072, "\r\n") -> (w2071:string)
            n1673 = VISA Write(VISA resource name=w2074, write buffer=w2071, error in (no error)=w2073) -> (VISA resource name out=w2078:refnum<visa-resource-name>, return count=w2075:u32, error out=w2077:errorcluster)
            n1674 = flat-sequence {
              tunnel: w2077 -> [w2080]
              tunnel: [w2080] -> w2076
              frame #0 {
                n1675 = local write "Due Write"("" ("Command")) -> ()
                n1676 = Wait (ms)(milliseconds to wait=u32 5) -> ()  [unwired: 1 out]
              }
            }
          }
        }
        "Port 2a" <- TRUE ("Port 2a")
      }
      frame Error {
        w2097 = u16 0 items=["None", "XON/XOFF", "RTS/CTS", "XON/XOFF & RTS/CTS", "DTR/DSR", "XON/XOFF & DTR/DSR"] ("flow control (0:none)  2")
        w2095 = u16 10 items=["1.0"=10, "1.5"=15, "2.0"=20] ("stop bits 2")
        w2093 = u16 0 items=["None", "Odd", "Even", "Mark", "Space"] ("parity 2")
        w2094 = u32 10000  # timeout (10sec)
        n1677 = VISA Clear(VISA resource name=w2089, error in (no error)=w2086) -> (VISA resource name out=w2088:refnum<visa-resource-name>, error out=w2087:errorcluster)
        n1678 = VISA Close(VISA resource name=w2088, error in (no error)=w2087) -> (error out=w2090:errorcluster)
        n1679 = call <vilib>:"Clear Errors.vi"("error in (no error)"=w2090) -> ()  [unwired: 5 in, 2 out]
        n1680 = local write "Port 2a"(FALSE ("Port 2a")) -> ()
        n1681 = local read "Com Port 2"() -> (w2083:refnum<visa-resource-name>)
        "visa due" <- w2083
        n1682 = call-poly "VISA Configure Serial Port"("VISA resource name"=w2083, "timeout (10sec)"=w2094, "baud rate (9600)"=u32 250000 ("baud rate  2"), "data bits (8)"=u16 8 ("data bits  2"), "parity (0:none)"=w2093, "stop bits (10: 1 bit)"=w2095, "flow control (0:none)"=w2097) -> ("VISA resource name out"=w2098:refnum<visa-resource-name>, "error out"=w2099:errorcluster)  [unwired: 7 in]
        n1683 = flat-sequence {
          tunnel: w2098 -> [w2101]
          tunnel: w2099 -> [w2100]
          tunnel: [w2101] -> w2091
          tunnel: [w2100] -> w2084
          frame #0 {
            n1684 = Wait (ms)(milliseconds to wait=u32 50) -> ()  [unwired: 1 out]
          }
        }
        "Residual Due" <- ""
      }
    }
    "error out 9" <- w2025
    n1685 = local read "Quit"() -> (w2027:bool)
    "Error Due" <- w2032
  }
  n1686 = local write "FRICVALZ"(0.0 ("FRICVALZ")) -> ()
  n1687 = property on="RUN" class="Bool (strict)"("Visible"=TRUE) -> ()  [unwired: 2 in, 2 out]
  n1688 = while {
    tunnel: [w2116] -> _
    tunnel: [w2103] -> w54
    i -> [w2116]
    stop <- w2103 stop-if-true
    n1689 = local read "conststatus"() -> (w2107:dbl)
    n1690 = local read "Main Tab"() -> (w2105:T2)
    n1691 = local read "EDIT"() -> (w2122:bool)
    n1692 = local read "Rate"() -> (w2121:dbl)
    n1693 = case shown="True" w2122 {
      tunnel: [FALSE TRUE] -> _
      frame False {
      }
      frame True {
      }
    }
    n1694 = Equal?(x=w2105, y=T28."About" ("Main Tab")) -> (x = y?=w2114:bool)
    n1695 = Equal?(x=w2107, y=0.0) -> (x = y?=w2108:bool)
    n1696 = Divide(x=1.0, y=w2121) -> (x/y=w2117:dbl)
    "Time 2" <- w2117
    n1697 = case shown="True" w2108 {
      frame False {
      }
      frame True {
        # "C:\\WinDucom\\calibrate WO 2391.dcf"
        n1698 = local write "Lan flag"(22) -> ()
        n1699 = local write "conststatus"(10.0 ("rpm value : 2")) -> ()
        n1700 = String To Path(string="C:\\LAB-IQ\\calibrate WO 2465.dcf") -> (path=w2128:path)
        n1701 = Open/Create/Replace File "Open File"(file path (use dialog)=w2128) -> (refnum out=w2126:refnum<file>)  [unwired: 5 in, 2 out]
        n1702 = for {
          N: 23 -> [_]
          tunnel: w2126 -> [w2137]
          i -> [w2131]
          (unwired) TRUE ("line mode (F)")
          n1703 = Read from Text File "Read File"(file (use dialog)=w2137) -> (text=w2136:string)  [unwired: 3 in, 3 out]
          n1704 = Match Pattern(string=w2136, regular expression="]") -> (after substring=w2134:string)  [unwired: 1 in, 3 out]
          n1705 = String Subset(string=w2136, offset (0)=5, length (rest)=10 ("length (rest)")) -> (substring=w2129:string)
          n1706 = Fract/Exp String To Number(string=w2129) -> (number=w2130:dbl)  [unwired: 3 in, 1 out]
          n1707 = Match Pattern(string=w2134, regular expression="-") -> (before substring=w2132:string)  [unwired: 1 in, 3 out]
          n1708 = case shown="10" w2131 {
            tunnel: w2130 -> [_ _ _ _ _ _ _ _ _ _ w2144 _ _ _ _ _ _ _ _ _ _ _ _ _]
            tunnel: w2132 -> [_ _ _ _ w2140 w2141 w2142 _ _ _ _ _ _ _ _ _ _ _ _ _ w2145 w2146 w2147 _]
            frame 0 {
            }
            frame 1 {
            }
            frame 2 {
            }
            frame 3 {
            }
            frame 4 {
              n1709 = local write "Com Port 1"(w2140) -> ()
            }
            frame 5 {
              n1710 = local write "Com Port 2"(w2141) -> ()
              n1711 = local write "visa due"(w2141) -> ()
            }
            frame 6 {
              n1712 = String To Path(string=w2142) -> (path=w2143:path)
              n1713 = local write "File Path"(w2143) -> ()
              "String" <- w2142
            }
            frame 7 {
            }
            frame 8 {
            }
            frame 9 {
            }
            frame 10 {
              n1714 = local write "Language Selection"(w2144) -> ()
            }
            frame 11 {
            }
            frame 12 {
            }
            frame 13 {
            }
            frame 14 {
            }
            frame 15 {
            }
            frame 16 {
            }
            frame 17 {
            }
            frame 18 {
            }
            frame 21 {
            }
            frame 22 {
              n1715 = local write "Com Port 3"(w2145) -> ()
            }
            frame 20 {
              n1716 = local write "Camera Port :"(w2146) -> ()
            }
            frame 19 {
              n1717 = local write "C3 :"(w2147) -> ()
            }
            frame 23, Default {
            }
          }
        }
      }
    }
    n1718 = Select(t=u32 2500 ("milliseconds to wait"), s=w2114, f=u32 500 ("milliseconds to wait")) -> (s? t:f=w2112:u32)
    n1719 = Multiply(x=w2117, y=w2112) -> (x*y=w2119:dbl)
    n1720 = call "Elapsed Time2"("Time Target (s)"=w2119, "Auto Reset"=TRUE) -> ("Time has Elapsed"=w2109:bool)  [unwired: 10 in, 7 out]
    n1721 = case shown="True" w2109 {
      frame False {
      }
      frame True {
        n1722 = stacked-sequence {
          frame #0 {
            # "DATA PROCESSING"
            # "115 mV/N"
            n1723 = local read "Sample Temperature"() -> (w2150:dbl)
            n1724 = local read "RH Numeric:"() -> (→"Humidity ( %RH )" →"Hum":dbl)
            n1725 = local read "FRICVALZ"() -> (w2167:dbl)
            n1726 = local read "Friction"() -> (w2153:dbl)
            n1727 = call <vilib>:"Mean PtByPt.vi"("x"=w2150, "sample length"=100) -> ("mean"=w2149:dbl)  [unwired: 2 in, 1 out]
            "TEMP 2" <- w2149
            "TEMP 3" <- w2149
            n1728 = Subtract(x=w2153, y=w2167) -> (x-y=w2162:dbl)
            "FF 2" <- w2162
            "FF 4" <- w2162
            n1729 = local read "Ambient Temperature"() -> (→"AIR TEMP":dbl)
            n1730 = local read "TEMP"() -> (w2166:dbl)
            n1731 = local write "FF 3"(w2162) -> ()
            n1732 = Compound Arithmetic op=OR("FRICVALZ 4", "FRICVALZ 3", "FRICVALZ 2") -> (w2158:bool)
            n1733 = case shown="True" w2158 {
              tunnel: w2153 -> [_ w2173]
              frame False {
              }
              frame True {
                w2172 = FALSE ("FRICVALZ")
                n1734 = local write "FRICVALZ 3"(w2172) -> ()
                n1735 = local write "FRICVALZ 2"(w2172) -> ()
                n1736 = local write "FRICVALZ 4"(w2172) -> ()
                "FRICVALZ" <- w2173
              }
            }
            n1737 = Not A Number/Path/Refnum?(number/path/refnum=w2166) -> (NaN/Path/Refnum?=w2165:bool)
            n1738 = Not A Number/Path/Refnum?(number/path/refnum=w2162) -> (NaN/Path/Refnum?=w2164:bool)
            n1739 = Divide(x=w2162, y=1.96) -> (x/y=w2159:dbl)
            n1740 = Compound Arithmetic op=OR(w2165, w2164) -> (w2163:bool)
            n1741 = Not A Number/Path/Refnum?(number/path/refnum=w2159) -> (NaN/Path/Refnum?=w2160:bool)
            n1742 = case shown="True" w2163 {
              frame False {
              }
              frame True {
                n1743 = local write "TEMP"(0.0 ("TEMP")) -> ()
                n1744 = local write "FF 2"(0.0 ("FF 2")) -> ()
                n1745 = local write "reinit"(TRUE ("reinit")) -> ()
              }
            }
            n1746 = local write "TEMP"(w2149) -> ()
            n1747 = Select(t=0.0, s=w2160, f=w2159) -> (s? t:f=w2152:dbl)
            "COF 2" <- w2152
            n1748 = local write "COF 3"(w2152) -> ()
          }
        }
      }
    }
    n1749 = Wait (ms)(milliseconds to wait=u32 50) -> ()  [unwired: 1 out]
    n1750 = local read "Quit"() -> (w2103:bool)
    "Rate" <- 2500.0 ("No of Samples")
  }
  n1751 = while {
    tunnel: [w2193] -> _
    tunnel: [w2176] -> w56
    tunnel: w1 -> [_]
    i -> [w2193]
    stop <- w2176 stop-if-true
    # "C:\\LAB-IQ-NXT\\Scar View.exe"
    n1752 = local read "OK Button 16"() -> (w2183:bool)
    n1753 = local read "Main Tab"() -> (w2177:T2)
    n1754 = local read "service 3"() -> (w2178:bool)
    n1755 = local read "OPEN 6"() -> (w2180:bool)
    n1756 = local read "EDIT 2"() -> (w2182:bool)
    n1757 = flat-sequence {
      frame #0 {
        n1758 = stacked-sequence {
          frame #0 {
            n1759 = local read "EDIT"() -> (w2671:bool)
            n1760 = case shown="False" w2671 {
              tunnel: [u8 2 ("Disabled") u8 0 ("Disabled")] -> _
              frame False {
                w2673 = FALSE
                n1761 = local write "Password"("") -> ()
                n1762 = local write "x = y?"(w2673) -> ()
                n1763 = property on="Password" class="Str"("Visible"=w2673) -> ()  [unwired: 2 in, 2 out]
              }
              frame True {
                n1764 = property on="Password" class="Str"("Visible"=TRUE) -> ()  [unwired: 2 in, 2 out]
              }
            }
            "dipl pwd" <- "@143$\n" ("dipl pwd")
          }
          frame #1 {
          }
          frame #2 {
          }
          frame #3 {
          }
          frame #4 {
            n1765 = String To Byte Array(string="Password") -> (unsigned byte array=w2684:u8[])
            n1766 = Search 1D Array(1D array=w2684, element=u8 10) -> (index of element=w2682:i32)  [unwired: 1 in]
            n1767 = Index Array(array=w2684, index=w2682) -> (element=w2683:u8)
            n1768 = Equal?(x=w2683, y=10) -> (x = y?=w2679:bool)
            n1769 = case shown="True" w2679 {
              frame False {
              }
              frame True {
                # "password"
                # "password"
                n1770 = local read "Password"() -> (w2696:string)
                n1771 = String To Byte Array(string=w2696) -> (unsigned byte array=w2699:u8[])
                n1772 = String To Byte Array(string="@143$\n") -> (unsigned byte array=w2686:u8[])
                n1773 = Array Size(array=w2699) -> (size(s)=w2695:i32)
                n1774 = Array Size(array=w2686) -> (size(s)=w2691:i32)
                n1775 = for {
                  N: w2695 -> [_]
                  tunnel: w2699 -> [w2712]
                  tunnel: [w2710] -> w2700 mode=indexing
                  tunnel: w2695 -> [w2707]
                  i -> [w2708]
                  n1776 = Decrement(x=w2707) -> (x-1=w2706:i32)
                  n1777 = Index Array(array=w2712, index=w2708) -> (element=w2711:u8)
                  n1778 = Equal?(x=w2708, y=w2706) -> (x = y?=w2705:bool)
                  n1779 = Number To Decimal String(number=w2711) -> (decimal integer string=w2709:string)  [unwired: 1 in]
                  n1780 = Select(t="", s=w2705, f="\r") -> (s? t:f=w2702:string)
                  n1781 = Concatenate Strings(w2709, w2702) -> (w2710:string)
                }
                n1782 = for {
                  N: w2691 -> [_]
                  tunnel: w2686 -> [w2723]
                  tunnel: [w2721] -> w2689 mode=indexing
                  tunnel: w2691 -> [w2718]
                  i -> [w2719]
                  n1783 = Decrement(x=w2718) -> (x-1=w2717:i32)
                  n1784 = Index Array(array=w2723, index=w2719) -> (element=w2722:u8)
                  n1785 = Equal?(x=w2719, y=w2717) -> (x = y?=w2716:bool)
                  n1786 = Number To Decimal String(number=w2722) -> (decimal integer string=w2720:string)  [unwired: 1 in]
                  n1787 = Select(t="", s=w2716, f="\r") -> (s? t:f=w2713:string)
                  n1788 = Concatenate Strings(w2720, w2713) -> (w2721:string)
                }
                n1789 = local read "file path"() -> (w2685:path)
                n1790 = call <vilib>:"Read Characters From File.vi"("file path (dialog if empty)"=w2685) -> ("character string"=w2698:string)  [unwired: 5 in, 3 out]
                "string" <- w2698
                n1791 = flat-sequence {
                  tunnel: [w2701] -> _
                  frame #0 {
                    w2701 = ""
                    n1792 = local write "Password"(w2701) -> ()
                  }
                }
                n1793 = Concatenate Strings(w2689) -> (w2690:string)
                n1794 = Concatenate Strings(w2698) -> (w2697:string)
                n1795 = Concatenate Strings(w2700) -> (w2693:string)
                n1796 = Equal?(x=w2693, y=w2697) -> (x = y?=w2688:bool)
                n1797 = Equal?(x=w2693, y=w2690) -> (x = y?=w2694:bool)
                n1798 = Or(x=w2688, y=w2694) -> (x .or. y?=→"x = y?":bool)
              }
            }
          }
        }
        n1799 = local read "x = y?"() -> (w2669:bool)
        n1800 = And(x="EDIT", y=w2669) -> (x .and. y?=w2667:bool)
        n1801 = case shown="True" w2667 {
          tunnel: [u8 2 ("Disabled") u8 0 ("Disabled")] -> w2666
          tunnel: [w2873 TRUE ("Visible")] -> w2665
          frame False {
            w2873 = FALSE ("Visible")
            n1802 = local write "EDIT 2"(w2873) -> ()
          }
          frame True {
          }
        }
        n1803 = case shown="True" "SAVE" {
          frame False {
          }
          frame True {
            n1804 = stacked-sequence {
              seq-local: [w2728 _ _] -> [_ w2869 _]
              frame #0 {
                w2724 = 0.0 ("number")
                w2725 = 0.0 ("number")
                (unwired) i16 5 ("precision (6)")
                # "[CH1]    - FF\n[CH2]   - TEMPERATURE\n[CH3]    - Humidity\n[CH4]    - AIR TEMP\n[CH5]\\- Visa Uno\n[CH6] \\- Visa Due\n[CH7]  \\- file path\n[CH8]   - Displacement Gain\n[CHA]   - Stroke Gain\n[CHB]   - Stroke PID Gain\n[CHC]   -Language Selection\n[CHD]   -Power +\n[CHE]   -Power_\n[CHF]   -Heater\n[CHG]   -Humidity Wet\n[CHH]   -Humidity Dry\n[CHI]   -Integral Time"
                n1805 = local read "Language Selection"() -> (w2771:enum16{"English", "Russian"})
                n1806 = Path To String(path="File Path") -> (string=w2787:string)
                n1807 = Number To Fractional String(number=w2724, width (-)=i16 10 ("precision (6)"), precision (6)=i16 5) -> (F-format string=w2778:string)  [unwired: 1 in]
                n1808 = Number To Fractional String(number=w2771, width (-)=i16 10 ("precision (6)"), precision (6)=i16 5) -> (F-format string=w2767:string)  [unwired: 1 in]
                n1809 = Number To Fractional String(number=w2725, width (-)=i16 10 ("precision (6)"), precision (6)=i16 5) -> (F-format string=w2761:string)  [unwired: 1 in]
                n1810 = Number To Fractional String(number=w2725, width (-)=i16 10 ("precision (6)"), precision (6)=i16 5) -> (F-format string=w2758:string)  [unwired: 1 in]
                n1811 = Number To Fractional String(number=w2725, width (-)=i16 10 ("precision (6)"), precision (6)=i16 5) -> (F-format string=w2753:string)  [unwired: 1 in]
                n1812 = Number To Fractional String(number=w2725, width (-)=i16 10 ("precision (6)"), precision (6)=i16 5) -> (F-format string=w2750:string)  [unwired: 1 in]
                n1813 = Number To Fractional String(number=w2725, width (-)=i16 10 ("precision (6)"), precision (6)=i16 5) -> (F-format string=w2745:string)  [unwired: 1 in]
                n1814 = local read "Com Port 1"() -> (w2727:refnum<visa-resource-name>)
                n1815 = local read "Com Port 2"() -> (w2726:refnum<visa-resource-name>)
                n1816 = Concatenate Strings(w2787, "\\" ("string")) -> (w2786:string)
                n1817 = Number To Fractional String(number=w2724, width (-)=i16 10 ("precision (6)"), precision (6)=i16 5) -> (F-format string=w2819:string)  [unwired: 1 in]
                n1818 = Number To Fractional String(number=w2724, width (-)=i16 10 ("precision (6)"), precision (6)=i16 5) -> (F-format string=w2818:string)  [unwired: 1 in]
                n1819 = Number To Fractional String(number=w2724, width (-)=i16 10 ("precision (6)"), precision (6)=i16 5) -> (F-format string=w2812:string)  [unwired: 1 in]
                n1820 = Number To Fractional String(number=w2724, width (-)=i16 10 ("precision (6)"), precision (6)=i16 5) -> (F-format string=w2806:string)  [unwired: 1 in]
                n1821 = Number To Fractional String(number=w2724, width (-)=i16 10 ("precision (6)"), precision (6)=i16 5) -> (F-format string=w2779:string)  [unwired: 1 in]
                n1822 = Concatenate Strings("[CHA]" ("string"), w2778, "- Stroke Gain" ("string"), "\r") -> (w2772:string)
                n1823 = Concatenate Strings("[CHC]" ("string"), w2767, "-Language Selection" ("string"), "\r") -> (w2764:string)
                n1824 = Concatenate Strings("[CHD]" ("string"), w2761, "-Power +" ("string"), "\r") -> (w2743:string)
                n1825 = Concatenate Strings("[CHG]" ("string"), w2750, "-Humidity Wet" ("string"), "\r") -> (w2740:string)
                n1826 = Concatenate Strings("[CHH]" ("string"), w2745, "-Humidity Dry" ("string"), "\r") -> (w2739:string)
                n1827 = Concatenate Strings("[CH1]" ("string"), w2819, " - FF" ("string"), "\r") -> (w2817:string)
                n1828 = Concatenate Strings("[CH2]" ("string"), w2818, " - TEMPERATURE" ("string"), "\r") -> (w2816:string)
                n1829 = Concatenate Strings("[CH3]" ("string"), w2812, " - Humidity" ("string"), "\r") -> (w2809:string)
                n1830 = Concatenate Strings("[CH4]" ("string"), w2806, " - AIR TEMP" ("string"), "\r") -> (w2802:string)
                n1831 = Concatenate Strings("[CH5]" ("string"), w2727, "- Visa Uno" ("string"), "\r") -> (w2795:string)
                n1832 = Concatenate Strings("[CH6]" ("string"), w2726, "- Visa Due" ("string"), "\r") -> (w2790:string)
                n1833 = Concatenate Strings("[CH7]" ("string"), w2786, "- file path" ("string"), "\r") -> (w2789:string)
                n1834 = Concatenate Strings("[CH8]" ("string"), w2779, "- Displacement Gain" ("string"), "\r") -> (w2782:string)
                n1835 = Concatenate Strings("[CHE]" ("string"), w2758, "-Power_" ("string"), "\r") -> (w2742:string)
                n1836 = Concatenate Strings("[CHF]" ("string"), w2753, "-Heater" ("string"), "\r") -> (w2741:string)
                n1837 = Concatenate Strings(w2817, w2816, w2809, w2802, w2795, w2790, w2789, w2782, w2772, w2764, w2743, w2742, w2741, w2740, w2739) -> (w2728:string)
                "gain" <- w2728
              }
              frame #1 {
                w2830 = 0.0 ("number")
                n1838 = local read "Camera Port :"() -> (w2833:string)
                n1839 = local read "C3 :"() -> (w2841:refnum<visa-resource-name>)
                n1840 = local read "Com Port 3"() -> (w2842:refnum<visa-resource-name>)
                n1841 = Concatenate Strings("[CH8]" ("string"), w2833, "- Visa Camera" ("string"), "\r") -> (w2832:string)
                n1842 = Concatenate Strings("[CH7]" ("string"), w2841, "- Visa Humidity" ("string"), "\r") -> (w2837:string)
                n1843 = Number To Fractional String(number=w2830, width (-)=i16 10 ("precision (6)"), precision (6)=i16 5) -> (F-format string=w2857:string)  [unwired: 1 in]
                n1844 = Concatenate Strings("[CHL]" ("string"), w2842, "- Visa humid" ("string"), "\r") -> (w2845:string)
                n1845 = Number To Fractional String(number=w2830, width (-)=i16 10 ("precision (6)"), precision (6)=i16 5) -> (F-format string=w2864:string)  [unwired: 1 in]
                n1846 = Concatenate Strings("[CHK]" ("string"), w2857, "-TEMP INTERCEPT" ("string"), "\r") -> (w2853:string)
                n1847 = Concatenate Strings("[SNO]" ("string"), "" ("string"), "-" ("string"), "\r") -> (w2850:string)
                n1848 = Concatenate Strings("[CHJ]" ("string"), w2864, "-AIR TEMP INTERCEPT" ("string"), "\r") -> (w2854:string)
                n1849 = String To Path(string="C:\\LAB-IQ\\calibrate WO 2465.dcf") -> (path=w2843:path)
                n1850 = Concatenate Strings(w2869, w2854, w2853, w2850, w2845, w2837, w2832) -> (w2868:string)
                n1851 = call <vilib>:"Write Characters To File.vi"("append to file? (new file:F)"=FALSE, "character string"=w2868, "file path (dialog if empty)"=w2843) -> ()  [unwired: 2 in, 1 out]
              }
              frame #2 {
                n1852 = local write "Lan flag"(0.0 ("Lan flag")) -> ()
                n1853 = local write "conststatus"(0.0 ("rpm value : 2")) -> ()
                n1854 = local write "SAVE"(FALSE ("OK Button 14")) -> ()
              }
            }
          }
        }
        n1855 = property on="EDIT 2" class="Bool (strict)"("Visible"=w2665) -> ()  [unwired: 2 in, 2 out]
        n1856 = property on="SAVE" class="Bool (strict)"("Visible"=w2665) -> ()  [unwired: 2 in, 2 out]
        n1857 = property on="visa due" class="CmbBox"("Disabled"=w2666) -> ()  [unwired: 2 in, 2 out]
        n1858 = property on="File Path" class="Path"("Disabled"=w2666) -> ()  [unwired: 2 in, 2 out]
        n1859 = property on="Language Selection" class="Enum (strict)"("Visible"=w2665) -> ()  [unwired: 2 in, 2 out]
        n1860 = property on="SPEED OUT:" class="DigNum (strict)"("Disabled"=w2666) -> ()  [unwired: 2 in, 2 out]
      }
    }
    n1861 = local read "RUN"() -> (w2192:bool)
    n1862 = local read "RUN"() -> (w2190:bool)
    n1863 = case shown="True" "EDIT 3" {
      frame False {
      }
      frame True {
        n1864 = local write "EDIT 3"(FALSE ("EDIT 3")) -> ()
        n1865 = local write "Main Tab"(T2."About" ("Main Tab")) -> ()
      }
    }
    n1866 = case shown="False" w2192 {
      frame False {
        n1867 = local read "stopT"() -> (w2880:bool)
        n1868 = case shown="True" w2880 {
          frame False {
          }
          frame True {
            n1869 = local write "stopT"(FALSE) -> ()
          }
        }
      }
      frame True {
        "stopT" <- TRUE
      }
    }
    n1870 = case shown="False" w2190 {
      frame False {
      }
      frame True {
      }
    }
    n1871 = case shown="True" w2182 {
      frame False {
        n1872 = property on="Password 2" class="Str"("Visible"=FALSE) -> ()  [unwired: 2 in, 2 out]
        n1873 = local write "Password 2"("" ("Password")) -> ()
      }
      frame True {
        n1874 = property on="Password 2" class="Str"("Visible"=TRUE) -> ()  [unwired: 2 in, 2 out]
        n1875 = Equal?(x="Password 2", y="HFRR1234") -> (x = y?=w2205:bool)
        n1876 = case shown="True" w2205 {
          tunnel: "Password 2" -> [w2208 _]
          frame False {
            n1877 = String Length(string=w2208) -> (length=w2209:i32)
            n1878 = Greater Than 0?(x=w2209) -> (x > 0?=w2207:bool)
            n1879 = case shown="False" w2207 {
              frame False {
                n1880 = property on="Password 2" class="Str"("Caption.Text"="Password (Advance Setting)") -> ()  [unwired: 2 in, 2 out]
              }
              frame True {
                n1881 = property on="Password 2" class="Str"("Caption.Text"="Incorrect Password!") -> ()  [unwired: 2 in, 2 out]
              }
            }
          }
          frame True {
            n1882 = local write "EDIT 2"(FALSE ("EDIT 2")) -> ()
            n1883 = local write "Password 2"("" ("Password")) -> ()
